vi "Cleanup.vi"(8 "error in (no error)":errorcluster, 11 "Caching in":refnum<class "Caching.lvclass">) -> (0 "error out":errorcluster)   [LabVIEW 2020, in "HTTP Server.lvlib" / "Caching.lvclass"]
uses:
  Caching.lvclass
  Caching.lvclass/Caching.ctl
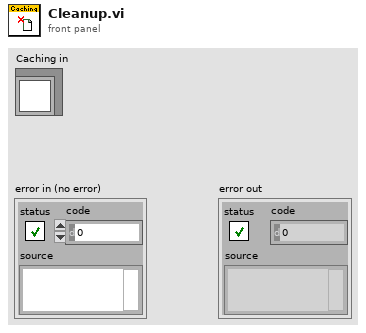
[diagram p1: front panel]
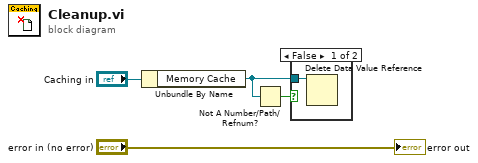
[diagram p0: block diagram]
diagram:
  n1 = Unbundle By Name("Caching in") -> ("Memory Cache"=w1:refnum<data-value>)
  n2 = Not A Number/Path/Refnum?(number/path/refnum=w1) -> (NaN/Path/Refnum?=w2:bool)
  n3 = case shown="False" w2 {
    tunnel: w1 -> [w5 _]
    frame False {
      n4 = Delete Data Value Reference(data value reference=w5) -> ()  [unwired: 1 in, 2 out]
    }
    frame True {
    }
  }
  "error out" <- "error in (no error)"
